vi "DisplayDataChartDialogGlobal.vi"(7 "Action":T1) -> ()   [LabVIEW 2012]
uses:
  DisplayDataChartDialogGlobalAction.ctl
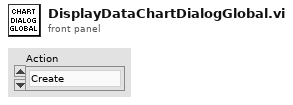
[diagram p1: front panel]
types:
  T1 = typedef "DisplayDataChartDialogGlobalAction.ctl" = enum16{"Create", "Close"}
  T2 = enum32{"Invalid", "Standard", "Closed", "Hidden", "Minimized", "Maximized"}
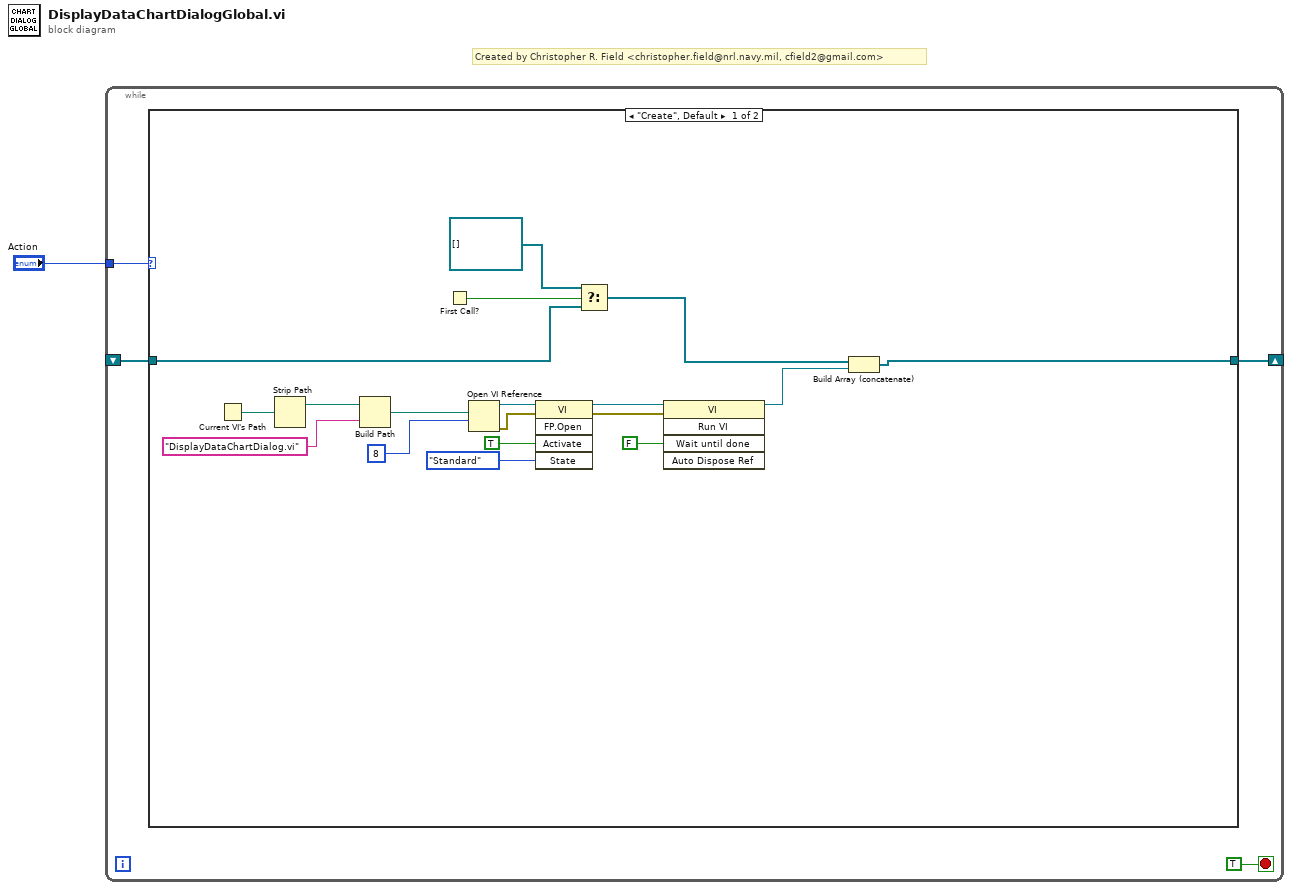
[diagram p0: block diagram]
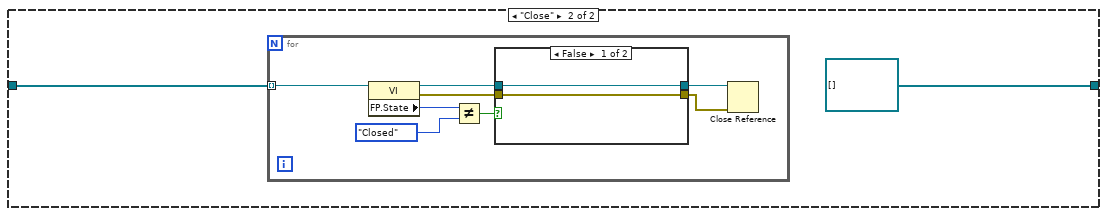
[diagram p2: hidden frame]
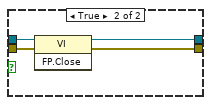
[diagram p3: hidden frame]
diagram:
  # "Created by Christopher R. Field <christopher.field@nrl.navy.mil, cfield2@gmail.com>"
  n1 = while {
    tunnel: "Action" -> [w4]
    shift-right: [w3] -> _
    shift-left: _ -> [w2]
    stop <- TRUE stop-if-true
    n2 = case shown="\"Create\", Default" w4 {
      tunnel: [w10 refnum<vi>[] []] -> w3
      tunnel: w2 -> [w7 w25]
      frame "Create", Default {
        n3 = Current VI's Path() -> (path=w23:path)
        n4 = Strip Path(path=w23) -> (stripped path=w22:path)  [unwired: 1 out]
        n5 = Build Path(base path=w22, name or relative path="DisplayDataChartDialog.vi") -> (appended path=w20:path)
        n6 = First Call?() -> (First Call?: T/F=w9:bool)
        n7 = Open VI Reference(vi path=w20, options=8) -> (vi reference=w18:refnum<vi>, error out=w17:errorcluster)  [unwired: 4 in]
        n8 = invoke class="VI" method="FP.Open"(reference=w18, error in=w17, "Activate"=TRUE ("Front Panel Window:Is Frontmost"), "State"=T2."Standard" ("Front Panel Window:State")) -> (reference out=w14:refnum<vi>, error out=w13:errorcluster)  [unwired: 1 in, 3 out]
        n9 = Select(t=refnum<vi>[] [], s=w9, f=w7) -> (s? t:f=w6:refnum<vi>[])
        n10 = invoke class="VI" method="Run VI"(reference=w14, error in=w13, "Wait until done"=FALSE ("Wait Until Done")) -> (reference out=w11:refnum<vi>)  [unwired: 2 in, 4 out]
        n11 = Build Array (concatenate)(w6, w11) -> (w10:refnum<vi>[])
      }
      frame "Close" {
        n12 = for {
          tunnel: w25 -> [w29] mode=indexing
          n13 = property class="VI"(reference=w29) -> (reference out=w31:refnum<vi>, error out=w28:errorcluster, "FP.State"=w33:T2)  [unwired: 1 in]
          n14 = Not Equal?(x=w33, y=T2."Closed") -> (x != y?=w30:bool)
          n15 = case shown="False" w30 {
            tunnel: w31 -> [w35 w39]
            tunnel: [w35 w38] -> w26
            tunnel: w28 -> [w34 w37]
            tunnel: [w34 w36] -> w27
            frame False {
            }
            frame True {
              n16 = invoke class="VI" method="FP.Close"(reference=w39, error in=w37) -> (reference out=w38:refnum<vi>, error out=w36:errorcluster)  [unwired: 1 in, 1 out]
            }
          }
          n17 = Close Reference(reference=w26, error in (no error)=w27) -> ()  [unwired: 1 out]
        }
      }
    }
  }
